vi "PQlistColumns.vi"(8 "error in":errorcluster, 10 "table":string, 11 "conn":u64) -> (0 "error out":errorcluster, 2 "Data":string[](array[string]), 3 "conn_out":u64)   [LabVIEW 2019, in "libpqutility64.lvlib"]
uses:
  libpqutility64.lvlib
  libpqlv64/src/PQgetResult.vi
  libpqlv64/src/PQclear.vi
  PQfetchTables.vi
  libpqlv64/src/PQresultErrorMessage.vi
  libpqlv64/src/PQresultStatus.vi
  libpqlv64/src/PQsendQuery.vi
  libpqlv64/src/PQgetvalue.vi
  libpqlv64/src/PQntuples.vi
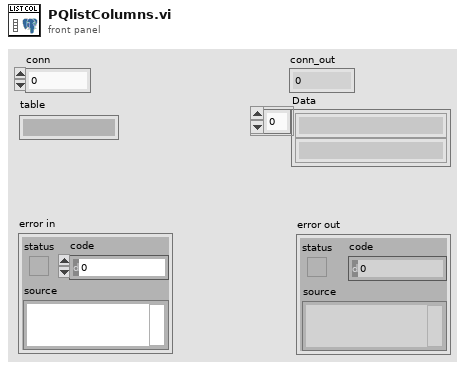
[diagram p1: front panel]
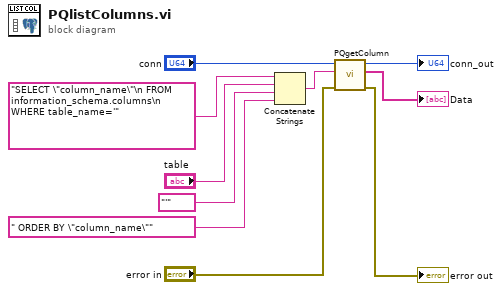
[diagram p0: block diagram]
diagram:
  n1 = Concatenate Strings("SELECT \"column_name\"\n FROM information_schema.columns\n WHERE table_name='" ("query"), "table", "'" ("query"), " ORDER BY \"column_name\"" ("query")) -> (w7:string)
  n2 = call "PQgetColumn.vi"("error in"="error in", "query"=w7, "conn"="conn") -> ("error out"=→"error out":errorcluster, "Data"=→"Data":string[], "conn_out"=→"conn_out":u64)  [unwired: 6 in]
